vi "ULxTaskInfo.vi"(0 "task in":refnum<k24>) -> (1 "NumberOfChannels":u32, 2 "Task":i32, 3 "ToString":string)   [LabVIEW 2010]
uses:
  C:/Program Files/National Instruments/LabVIEW 2010/vi.lib/ULx/ULx_LV.dll
  Program Files/National Instruments/LabVIEW 2010/vi.lib/ULx/ULx_LV.dll
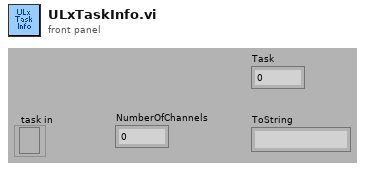
[diagram p1: front panel]
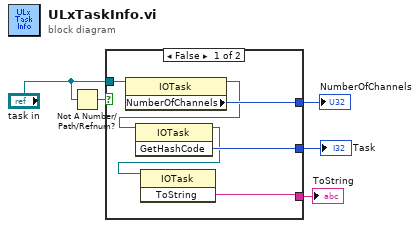
[diagram p0: block diagram]
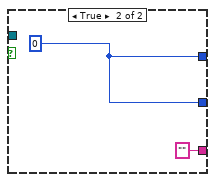
[diagram p2: hidden frame]
diagram:
  n1 = Not A Number/Path/Refnum?(number/path/refnum="task in") -> (NaN/Path/Refnum?=w4:bool)
  n2 = case shown="False" w4 {
    tunnel: "task in" -> [w11 _]
    tunnel: [w10 w13] -> w5
    tunnel: [w8 w13] -> w2
    tunnel: [w6 "" ("ToString")] -> w1
    frame False {
      n3 = property class="IOTask"(reference=w11) -> (reference out=w9:refnum<k24>, "NumberOfChannels"=w10:u32)  [unwired: 1 in, 1 out]
      n4 = invoke class="IOTask" method="GetHashCode"(reference=w9) -> (reference out=w7:refnum<k24>, "GetHashCode"=w8:i32)  [unwired: 2 in, 1 out]
      n5 = invoke class="IOTask" method="ToString"(reference=w7) -> ("ToString"=w6:string)  [unwired: 2 in, 2 out]
    }
    frame True {
      w13 = 0 ("NumberOfChannels")
    }
  }
  "NumberOfChannels" <- w5
  "Task" <- w2
  "ToString" <- w1
